vi "mcc data transfer processing.vi"(9 "s? t:f":dbl[](array[numeric]), 10 "Crew Status":bool[](array[boolean])) -> (0 "P2":string, 1 "P1":string, 2 "H":string, 3 "N":string, 4 "output cluster":T1, 5 "appended array":string[](array[string]))   [LabVIEW 2021]
panel:
  out "result":i32
  out "concatenated string":string
  out "timed out?":bool
  out "unsigned byte array 2":u8[](array[numeric])
  out "JSON string":string
  out "notification":dbl[](array[numeric])
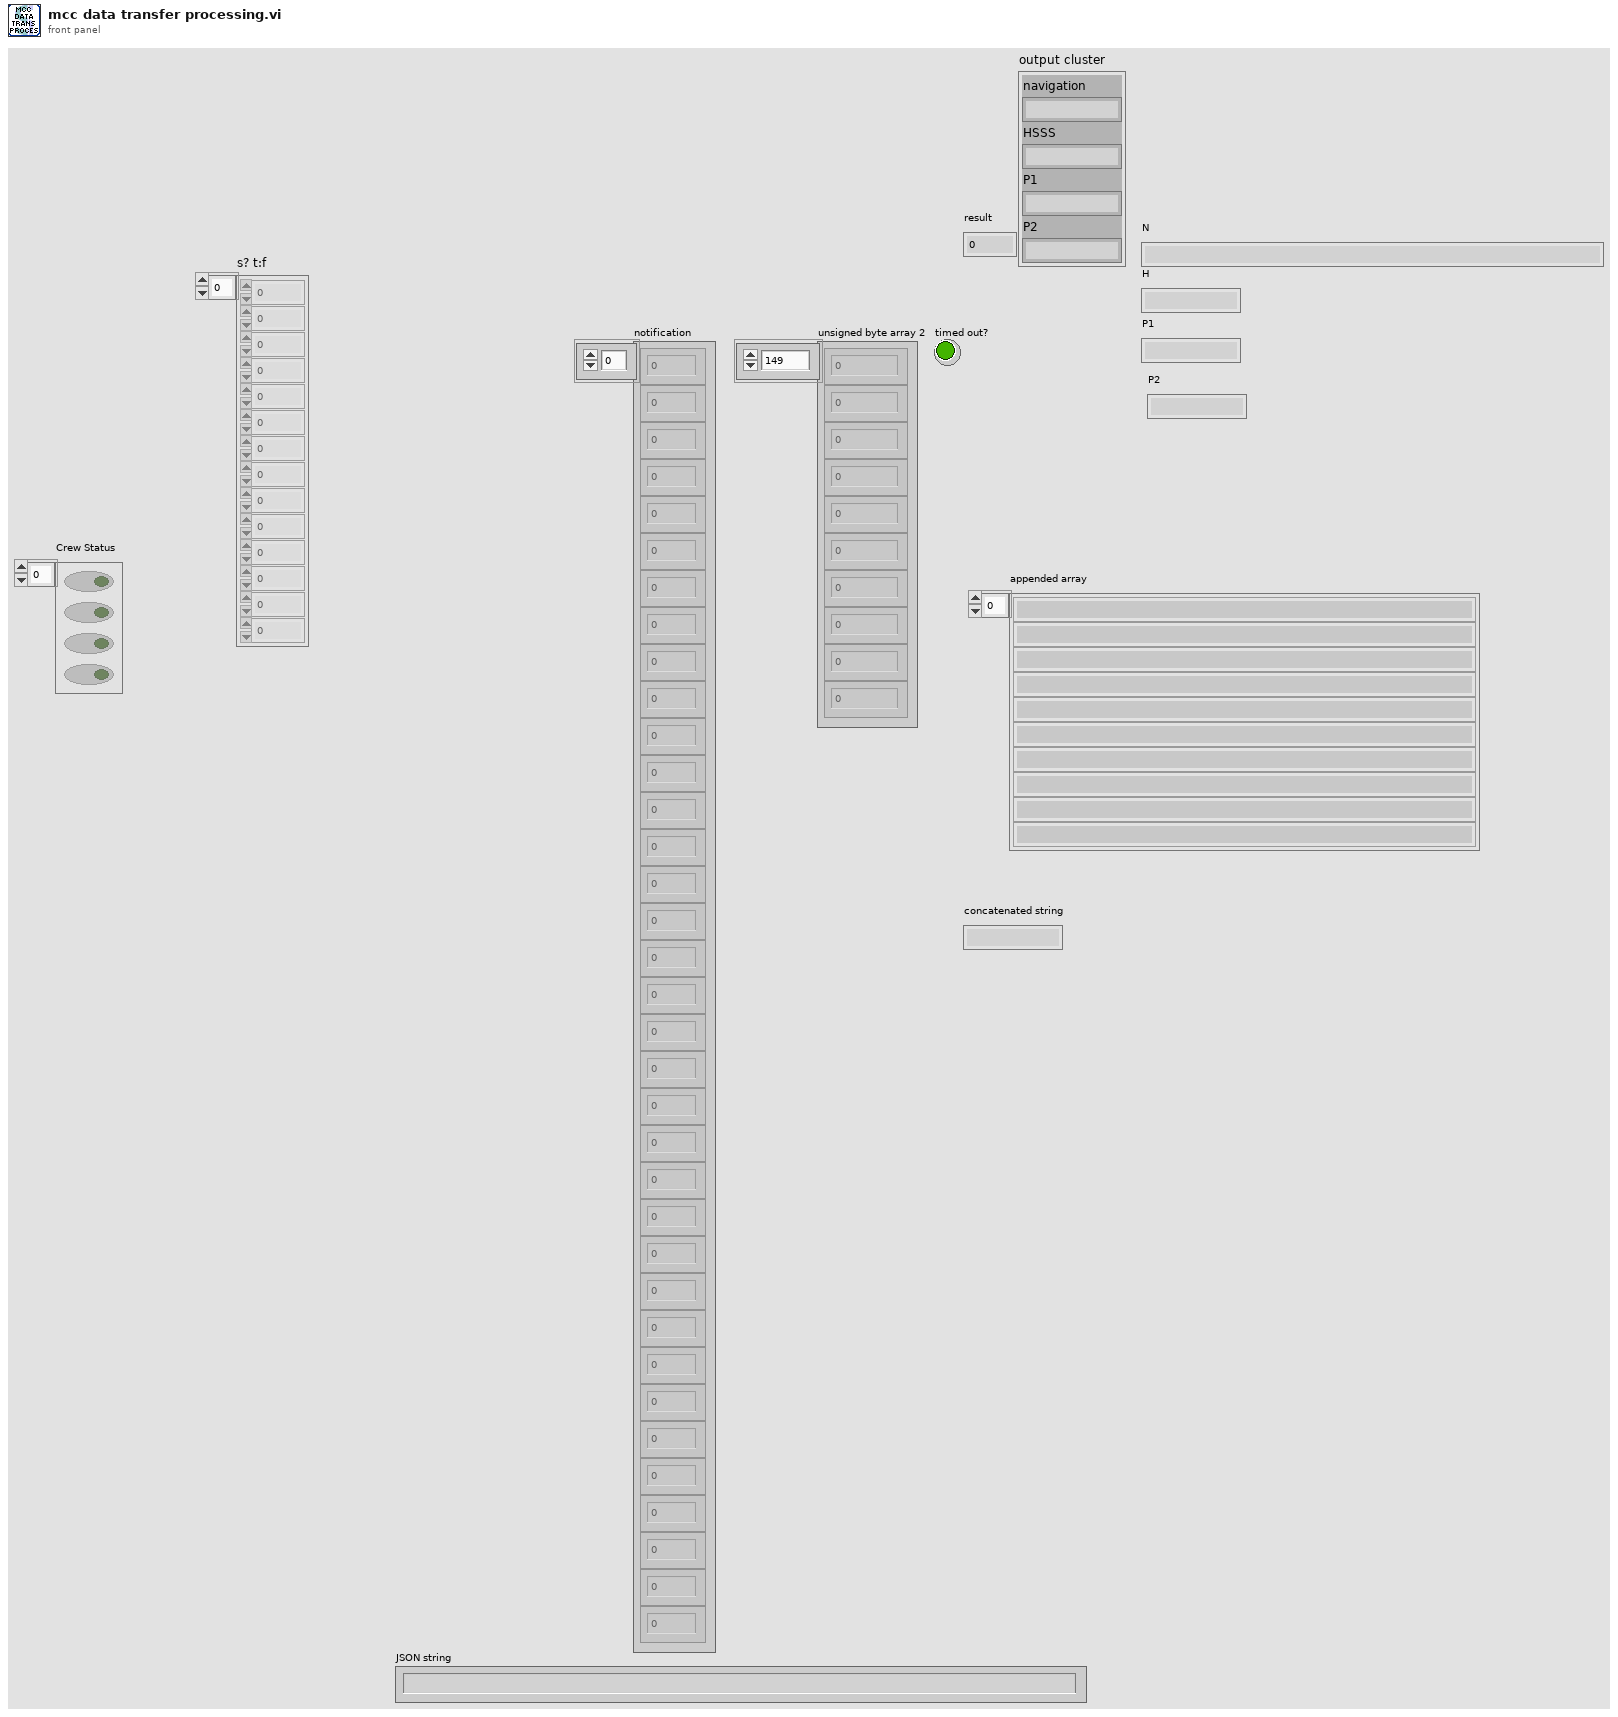
[diagram p1: front panel]
types:
  T1 = cluster{"navigation":string, "HSSS":string, "P1":string, "P2":string}
  T2 = typedef "LVDateTimeRec.ctl" = cluster{"fractional second":dbl, "second":i32, "minute":i32, "hour":i32, "day of month":i32, "month":i32, "year":i32, "day of week":i32, "day of year":i32, "DST":i32}
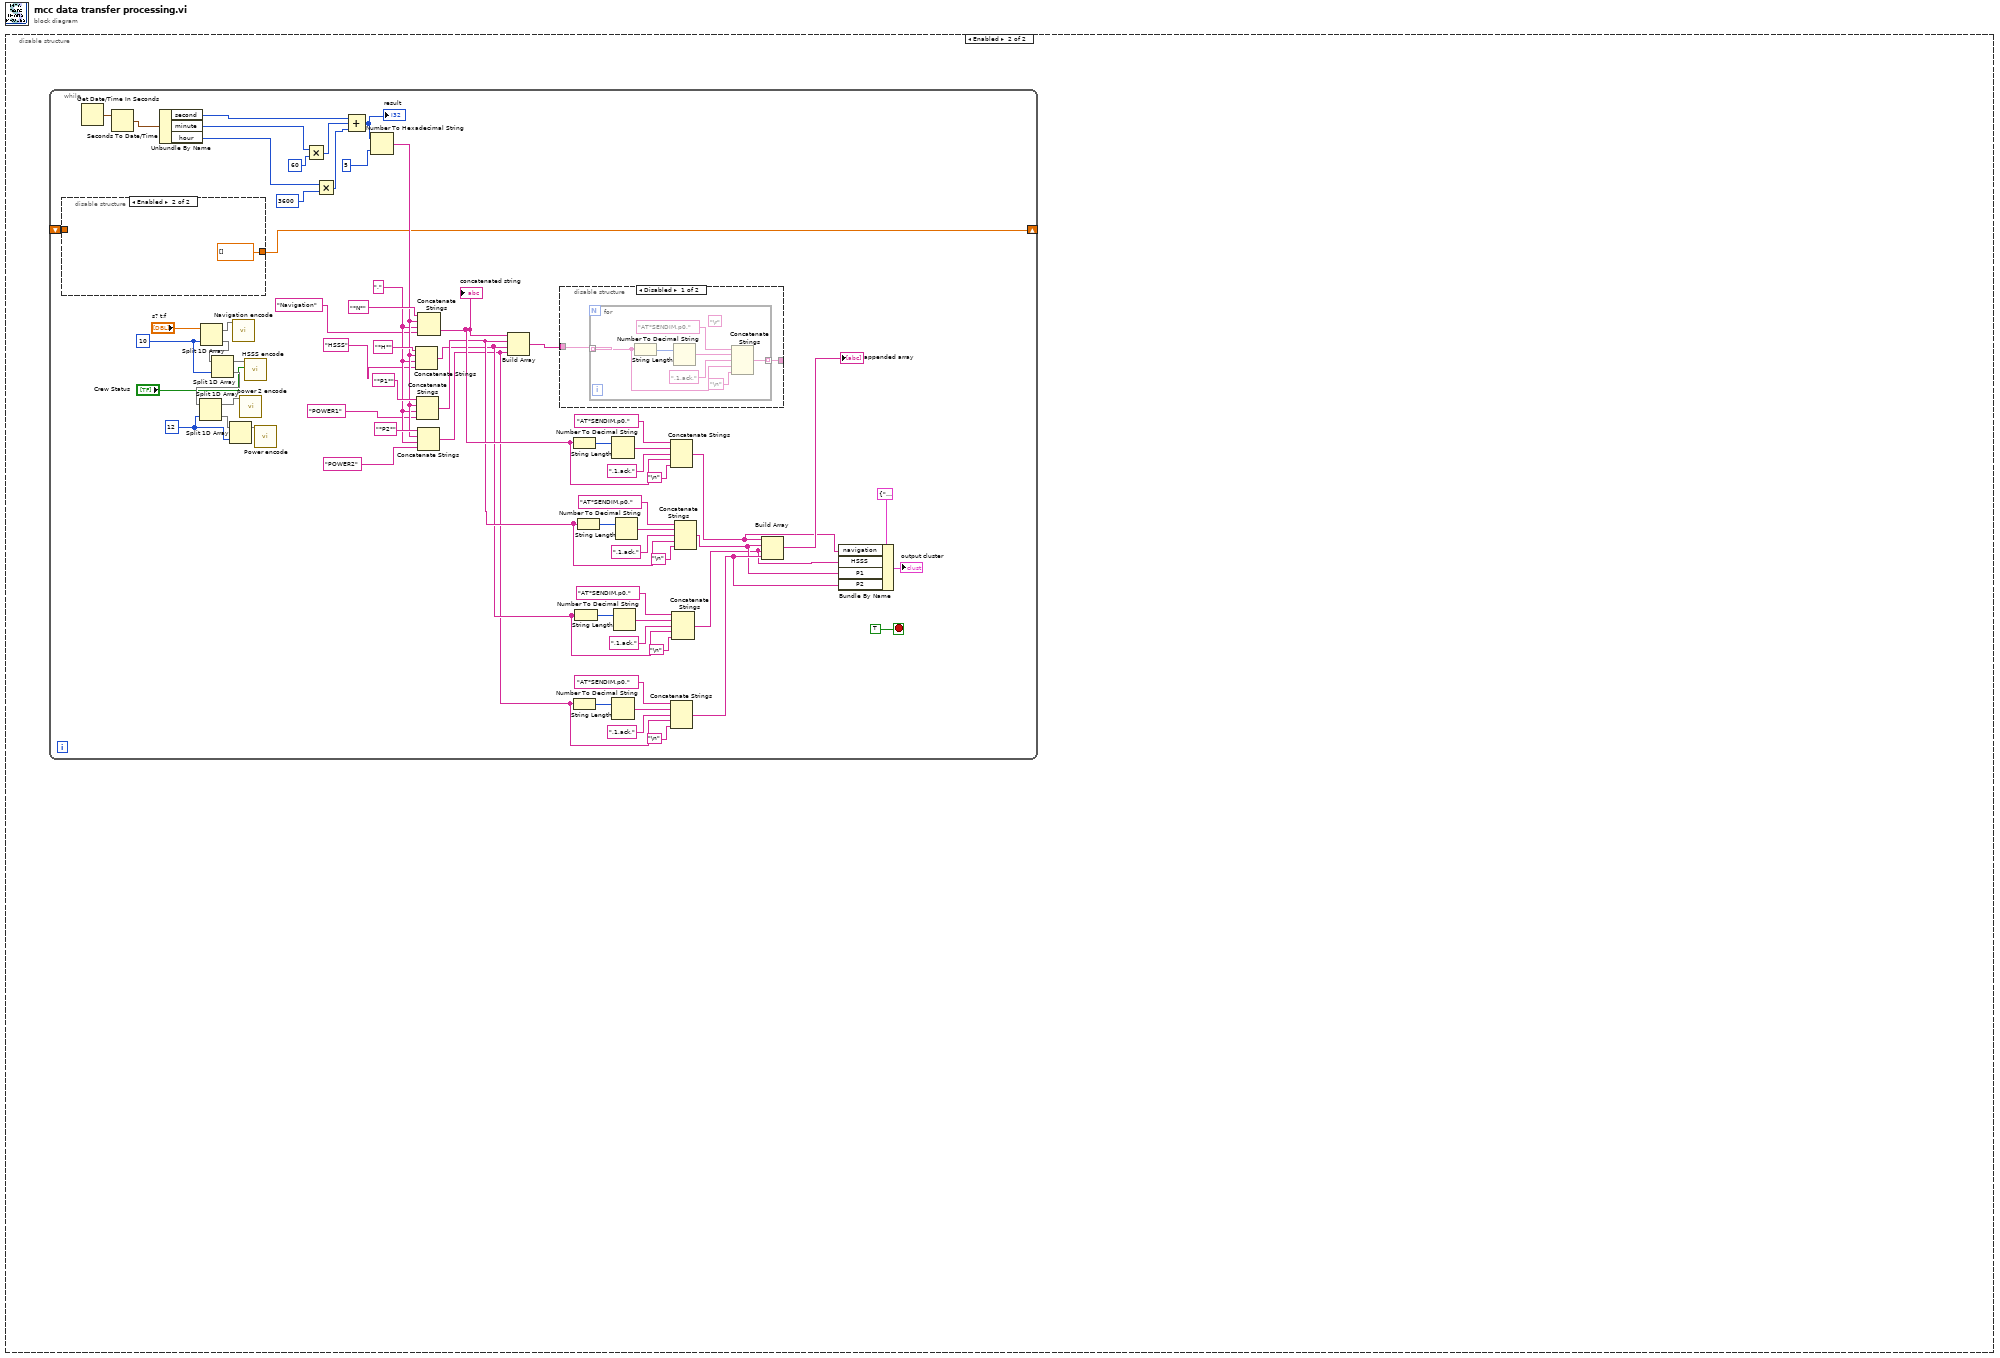
[diagram p0: block diagram]
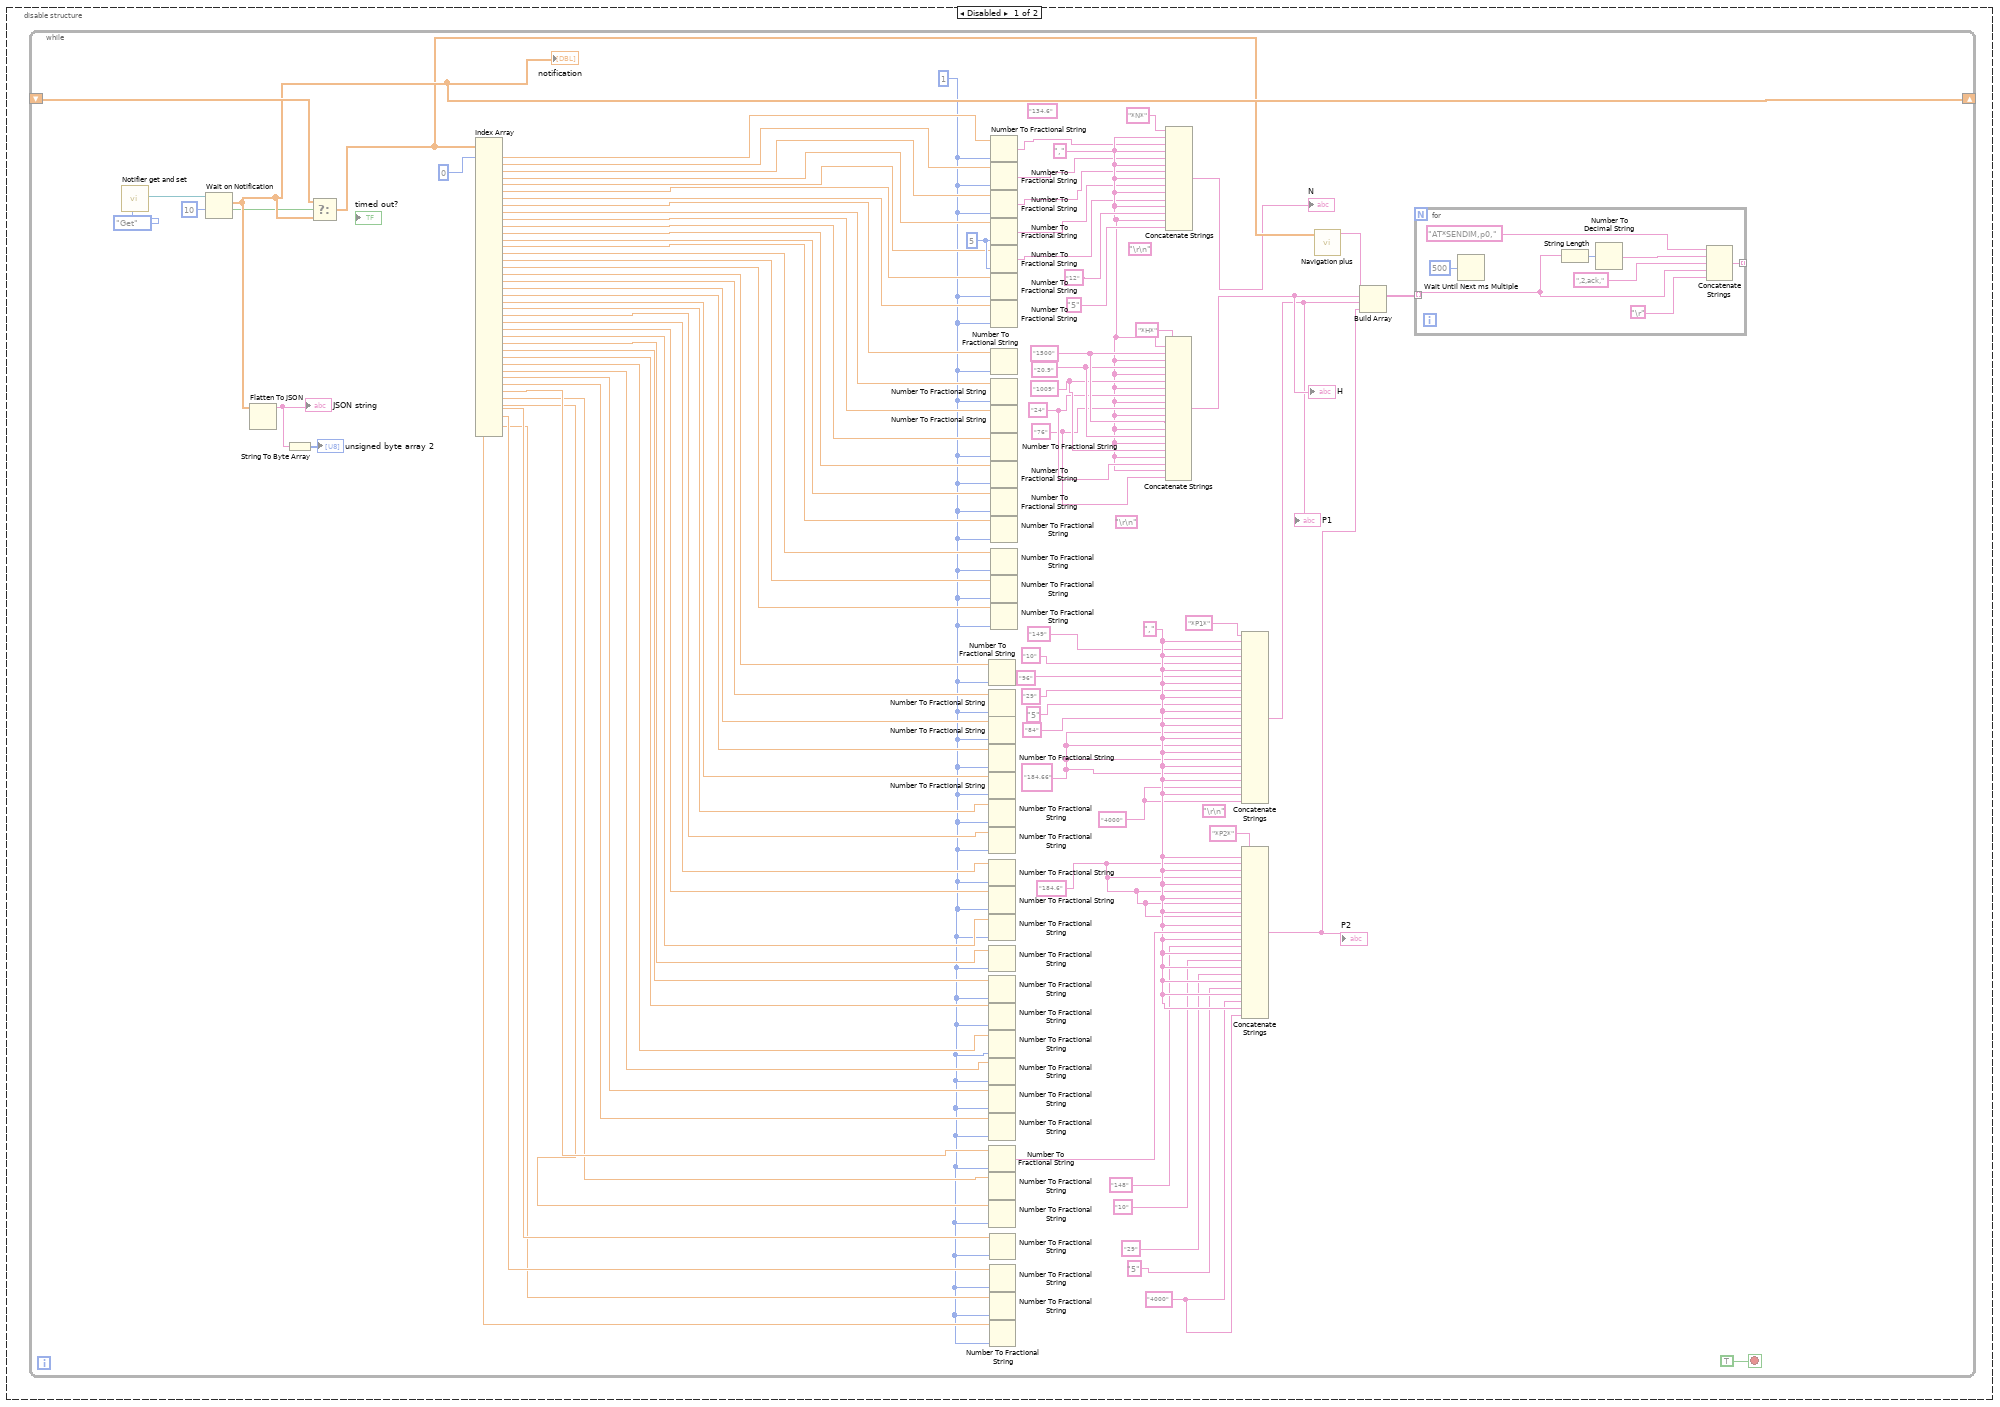
[diagram p2: hidden frame]
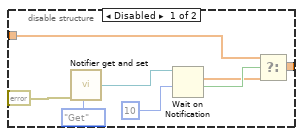
[diagram p4: hidden frame]
diagram:
  n1 = disable-structure shown="Enabled" {
    frame Disabled {
      n2 = while {
        shift-right: [w45] -> _
        shift-left: _ -> [w46]
        stop <- TRUE stop-if-true
        w15 = "184.6" ("string")
        w16 = "184.66" ("string")
        (unwired) "134.6" ("string")
        w28 = "4000"
        w29 = "4000"
        w32 = "76"
        w33 = "24"
        w34 = "1009" ("string")
        w35 = "20.9" ("string")
        w36 = "1500" ("string")
        (unwired) "\r\n"
        w40 = ","
        (unwired) "\r\n"
        w92 = i16 5 ("width (-)")
        w44 = i16 1 ("width (-)")
        (unwired) "\r\n"
        w17 = "," ("string")
        n3 = call "Notifier get and set.vi"("Operation"=enum16{"Init", "Get", "Set"}."Get") -> ("notifier out"=w5:refnum<notifier>)  [unwired: 9 in, 1 out]
        n4 = Wait on Notification(notifier=w5, timeout in ms (-1)=10) -> (notification=w45:dbl[], timed out?=w4:bool)  [unwired: 2 in, 2 out]
        "notification" <- w45
        n5 = Flatten To JSON(anything=w45) -> (JSON string=w7:string)  [unwired: 2 in, 1 out]
        "JSON string" <- w7
        n6 = String To Byte Array(string=w7) -> (unsigned byte array=→"unsigned byte array 2":u8[])
        n7 = Select(t=w46, s=w4, f=w45) -> (s? t:f=w3:dbl[])
        n8 = Index Array(array=w3, index #1=0 ("index")) -> (element #1=w90:dbl, element #2=w89:dbl, element #3=w88:dbl, element #4=w87:dbl, element #5=w86:dbl, element #6=w85:dbl, element #7=w84:dbl, element #8=w83:dbl, element #9=w82:dbl, element #10=w81:dbl, element #11=w80:dbl, element #12=w79:dbl, element #13=w78:dbl, element #14=w77:dbl, element #15=w76:dbl, element #16=w75:dbl, element #17=w74:dbl, element #18=w71:dbl, element #19=w70:dbl, element #20=w69:dbl, element #21=w68:dbl, element #22=w67:dbl, element #23=w66:dbl, element #24=w65:dbl, element #25=w64:dbl, element #26=w63:dbl, element #27=w62:dbl, element #28=w61:dbl, element #29=w60:dbl, element #30=w59:dbl, element #31=w58:dbl, element #32=w57:dbl, element #33=w56:dbl, element #34=w55:dbl, element #35=w54:dbl, element #36=w53:dbl, element #37=w52:dbl, element #38=w51:dbl, element #39=w50:dbl, element #40=w49:dbl, element #41=w48:dbl)  [unwired: 40 in]
        n9 = Number To Fractional String(number=w71, precision (6)=w44) -> ()  [unwired: 2 in, 1 out]
        n10 = Number To Fractional String(number=w70, precision (6)=w44) -> ()  [unwired: 2 in, 1 out]
        n11 = Number To Fractional String(number=w69, precision (6)=w44) -> ()  [unwired: 2 in, 1 out]
        n12 = Number To Fractional String(number=w68, precision (6)=w44) -> ()  [unwired: 2 in, 1 out]
        n13 = Number To Fractional String(number=w67, precision (6)=w44) -> ()  [unwired: 2 in, 1 out]
        n14 = Number To Fractional String(number=w66, precision (6)=w44) -> ()  [unwired: 2 in, 1 out]
        n15 = Number To Fractional String(number=w65, precision (6)=w44) -> ()  [unwired: 2 in, 1 out]
        n16 = Number To Fractional String(number=w64, precision (6)=w44) -> ()  [unwired: 2 in, 1 out]
        n17 = Number To Fractional String(number=w63, precision (6)=w44) -> ()  [unwired: 2 in, 1 out]
        n18 = Number To Fractional String(number=w62, precision (6)=w44) -> ()  [unwired: 2 in, 1 out]
        n19 = Number To Fractional String(number=w61, precision (6)=w44) -> ()  [unwired: 2 in, 1 out]
        n20 = Number To Fractional String(number=w60, precision (6)=w44) -> ()  [unwired: 2 in, 1 out]
        n21 = Number To Fractional String(number=w59, precision (6)=w44) -> ()  [unwired: 2 in, 1 out]
        n22 = Number To Fractional String(number=w58, precision (6)=w44) -> ()  [unwired: 2 in, 1 out]
        n23 = Number To Fractional String(number=w57, precision (6)=w44) -> ()  [unwired: 2 in, 1 out]
        n24 = Number To Fractional String(number=w56, precision (6)=w44) -> ()  [unwired: 2 in, 1 out]
        n25 = Number To Fractional String(number=w55, precision (6)=w44) -> ()  [unwired: 2 in, 1 out]
        n26 = Number To Fractional String(number=w54, precision (6)=w44) -> (F-format string=w43:string)  [unwired: 2 in]
        n27 = Number To Fractional String(number=w53) -> ()  [unwired: 3 in, 1 out]
        n28 = Number To Fractional String(number=w52, precision (6)=w44) -> ()  [unwired: 2 in, 1 out]
        n29 = Number To Fractional String(number=w51, precision (6)=w44) -> ()  [unwired: 2 in, 1 out]
        n30 = Number To Fractional String(number=w50, precision (6)=w44) -> ()  [unwired: 2 in, 1 out]
        n31 = Number To Fractional String(number=w49, precision (6)=w44) -> ()  [unwired: 2 in, 1 out]
        n32 = Number To Fractional String(number=w48, precision (6)=w44) -> ()  [unwired: 2 in, 1 out]
        n33 = Number To Fractional String(number=w90, precision (6)=w44) -> (F-format string=w14:string)  [unwired: 2 in]
        n34 = Number To Fractional String(number=w89, precision (6)=w44) -> (F-format string=w13:string)  [unwired: 2 in]
        n35 = Number To Fractional String(number=w88, precision (6)=w44) -> (F-format string=w12:string)  [unwired: 2 in]
        n36 = Number To Fractional String(number=w87, precision (6)=w92) -> (F-format string=w11:string)  [unwired: 2 in]
        n37 = Number To Fractional String(number=w86, precision (6)=w92) -> (F-format string=w10:string)  [unwired: 2 in]
        n38 = Number To Fractional String(number=w85, precision (6)=w44) -> ()  [unwired: 2 in, 1 out]
        n39 = Number To Fractional String(number=w84, precision (6)=w44) -> ()  [unwired: 2 in, 1 out]
        n40 = Number To Fractional String(number=w83, precision (6)=w44) -> ()  [unwired: 2 in, 1 out]
        n41 = Number To Fractional String(number=w82, precision (6)=w44) -> ()  [unwired: 2 in, 1 out]
        n42 = Number To Fractional String(number=w81) -> ()  [unwired: 3 in, 1 out]
        n43 = Number To Fractional String(number=w80, precision (6)=w44) -> ()  [unwired: 2 in, 1 out]
        n44 = Number To Fractional String(number=w79, precision (6)=w44) -> ()  [unwired: 2 in, 1 out]
        n45 = Number To Fractional String(number=w78, precision (6)=w44) -> ()  [unwired: 2 in, 1 out]
        n46 = Number To Fractional String(number=w77, precision (6)=w44) -> ()  [unwired: 2 in, 1 out]
        n47 = Number To Fractional String(number=w76, precision (6)=w44) -> ()  [unwired: 2 in, 1 out]
        n48 = Number To Fractional String(number=w75, precision (6)=w44) -> ()  [unwired: 2 in, 1 out]
        n49 = Number To Fractional String(number=w74, precision (6)=w44) -> ()  [unwired: 2 in, 1 out]
        n50 = Concatenate Strings("*H*" ("string"), w17, w36, w17, w35, w17, w34, w17, w33, w17, w32, w17, w36, w17, w35, w17, w34, w17, w33, w17, w32) -> (w73:string)
        "H" <- w73
        n51 = Concatenate Strings("*N*" ("string"), w17, w14, w17, w13, w17, w12, w17, w11, w17, w10, w17, "12", w17, "5") -> (→"N":string)
        n52 = Concatenate Strings("*P1*" ("string"), w40, "149" ("string"), w40, "10" ("string"), w40, "96" ("string"), w40, "29" ("string"), w40, "5" ("string"), w40, "84" ("string"), w40, w16, w40, w16, w40, w16, w40, w16, w40, w28, w40, w28) -> (w72:string)
        "P1" <- w72
        n53 = Concatenate Strings("*P2*" ("string"), w40, w15, w40, w15, w40, w15, w40, w15, w40, w15, w40, w43, w40, "148" ("string"), w40, "10" ("string"), w40, "29" ("string"), w40, "5" ("string"), w40, w29, w40, w29) -> (w37:string)
        "P2" <- w37
        n54 = call "Navigation plus.vi"("Array"=w3) -> ("String"=w1:string)  [unwired: 9 in, 1 out]
        n55 = Build Array(w1, w73, w72, w37) -> (w38:string[])
        n56 = for {
          tunnel: w38 -> [w96] mode=indexing
          tunnel: [w95] -> _ mode=indexing
          n57 = Wait Until Next ms Multiple(millisecond multiple=u32 500) -> ()  [unwired: 1 out]
          n58 = String Length(string=w96) -> (length=w99:i32)
          n59 = Number To Decimal String(number=w99) -> (decimal integer string=w98:string)  [unwired: 1 in]
          n60 = Concatenate Strings("AT*SENDIM,p0," ("string"), w98, ",2,ack," ("string"), w96, "\r") -> (w95:string)
        }
      }
    }
    frame Enabled {
      n61 = while {
        shift-right: [w148] -> _
        shift-left: _ -> [w149]
        stop <- TRUE stop-if-true
        w144 = 12 ("index")
        w141 = 10 ("index")
        w150 = ","
        n62 = disable-structure shown="Enabled" {
          disable-tunnel: w149 -> [w182 _]
          disable-tunnel: [w179 dbl[] [] ("initialized array")] -> w148
          frame Disabled {
            n63 = call "Notifier get and set.vi"("Operation"=enum16{"Init", "Get", "Set"}."Get", "error in"=errorcluster {"status"=FALSE, "code"=0, "source"=""}) -> ("notifier out"=w184:refnum<notifier>)  [unwired: 8 in, 1 out]
            n64 = Wait on Notification(notifier=w184, timeout in ms (-1)=10) -> (notification=w181:dbl[], timed out?=w183:bool)  [unwired: 2 in, 2 out]
            n65 = Select(t=w182, s=w183, f=w181) -> (s? t:f=w179:dbl[])
          }
          frame Enabled {
          }
        }
        n66 = Get Date/Time In Seconds() -> (seconds since 1Jan1904=w159:timestamp)
        n67 = Seconds To Date/Time(time stamp (now)=w159) -> (date time rec=w160:T2)  [unwired: 1 in]
        n68 = Unbundle By Name(w160) -> ("second"=w161:i32, "minute"=w162:i32, "hour"=w164:i32)
        n69 = Split 1D Array(array="s? t:f", index=w141) -> (first subarray=w143:dbl[], second subarray=w147:dbl[])
        n70 = Split 1D Array(array=w147, index=w141) -> (first subarray=w140:dbl[], second subarray=w146:dbl[])
        n71 = Split 1D Array(array=w146, index=w144) -> (first subarray=w139:dbl[], second subarray=w145:dbl[])
        n72 = Split 1D Array(array=w145, index=w144) -> (first subarray=w142:dbl[])  [unwired: 1 out]
        n73 = call "Navigation encode.vi"("Array"=w143) -> ()  [unwired: 10 in, 1 out]
        n74 = call "power 2 encode.vi"("Array"=w139) -> ()  [unwired: 10 in, 1 out]
        n75 = call "HSSS encode.vi"("Crew Status"="Crew Status", "Array"=w140) -> ()  [unwired: 9 in, 1 out]
        n76 = call "Power encode.vi"("Array"=w142) -> ()  [unwired: 10 in, 1 out]
        n77 = Multiply(x=w162, y=60) -> (x*y=w163:i32)
        n78 = Multiply(x=w164, y=3600) -> (x*y=w165:i32)
        n79 = Compound Arithmetic op=ADD(w161, w163, w165) -> (w166:i32)
        "result" <- w166
        n80 = Number To Hexadecimal String(1:i16 5 ("width (-)"), 2:w166) -> (0:w151:string)
        n81 = Concatenate Strings("*H*" ("string"), w151, w150, "HSSS" ("string")) -> (w110:string)
        n82 = Concatenate Strings("*P1*" ("string"), w151, w150, "POWER1" ("string")) -> (w111:string)
        n83 = Concatenate Strings("*P2*" ("string"), w151, w150, "POWER2" ("string")) -> (w109:string)
        n84 = Concatenate Strings("*N*" ("string"), w151, w150, "Navigation" ("string")) -> (w112:string)
        "concatenated string" <- w112
        n85 = Build Array(w112, w111, w110, w109) -> (w167:string[])
        n86 = disable-structure shown="Disabled" {
          disable-tunnel: w167 -> [w170 _]
          disable-tunnel: [w169 _] -> _
          frame Disabled {
            n87 = for {
              tunnel: w170 -> [w172] mode=indexing
              tunnel: [w173] -> w169 mode=indexing
              (unwired) "\r"
              n88 = String Length(string=w172) -> (length=w175:i32)
              n89 = Number To Decimal String(number=w175) -> (decimal integer string=w174:string)  [unwired: 1 in]
              n90 = Concatenate Strings("AT*SENDIM,p0," ("string"), w174, ",1,ack," ("string"), w172, "\n") -> (w173:string)
            }
          }
          frame Enabled {
          }
        }
        n91 = String Length(string=w112) -> (length=w130:i32)
        n92 = String Length(string=w109) -> (length=w115:i32)
        n93 = String Length(string=w110) -> (length=w120:i32)
        n94 = String Length(string=w111) -> (length=w125:i32)
        n95 = Number To Decimal String(number=w130) -> (decimal integer string=w129:string)  [unwired: 1 in]
        n96 = Number To Decimal String(number=w115) -> (decimal integer string=w114:string)  [unwired: 1 in]
        n97 = Number To Decimal String(number=w120) -> (decimal integer string=w119:string)  [unwired: 1 in]
        n98 = Number To Decimal String(number=w125) -> (decimal integer string=w124:string)  [unwired: 1 in]
        n99 = Concatenate Strings "Concatenate Strings"("AT*SENDIM,p0," ("string"), w129, ",1,ack," ("string"), w112, "\n") -> (w106:string)
        n100 = Concatenate Strings("AT*SENDIM,p0," ("string"), w114, ",1,ack," ("string"), w109, "\n") -> (w105:string)
        n101 = Concatenate Strings("AT*SENDIM,p0," ("string"), w119, ",1,ack," ("string"), w110, "\n") -> (w102:string)
        n102 = Concatenate Strings("AT*SENDIM,p0," ("string"), w124, ",1,ack," ("string"), w111, "\n") -> (w103:string)
        n103 = Build Array(w106, w103, w102, w105) -> (→"appended array":string[])
        n104 = Bundle By Name(cluster=T1 {"navigation"="", "HSSS"="", "P1"="", "P2"=""}, "navigation"=w106, "HSSS"=w102, "P1"=w103, "P2"=w105) -> (→"output cluster":T1)
      }
    }
  }
